vi "Read configuration.vi"(8 "error in":errorcluster, 11 "Multiplexer editor node in":refnum<class "Multiplexer editor node.lvclass">) -> (0 "error out":errorcluster, 2 "configuration":refnum<class "NISE_CEF_serializable configuration.lvclass">, 3 "Multiplexer editor node out":refnum<class "Multiplexer editor node.lvclass">)   [LabVIEW 2021, in "Multiplexer editor node.lvclass"]
uses:
  Multiplexer editor node.lvclass
  <vilib>/NI/Configuration Framework/serializable configuration/NISE_CEF_serializable configuration.lvclass
  Multiplexer editor node.lvclass/Multiplexer editor node.ctl
  configuration/Multiplexer configuration.lvclass
  C:/Program Files (x86)/National Instruments/LabVIEW 2021/vi.lib/NI/Configuration Framework/serializable configuration/NISE_CEF_serializable configuration.lvclass
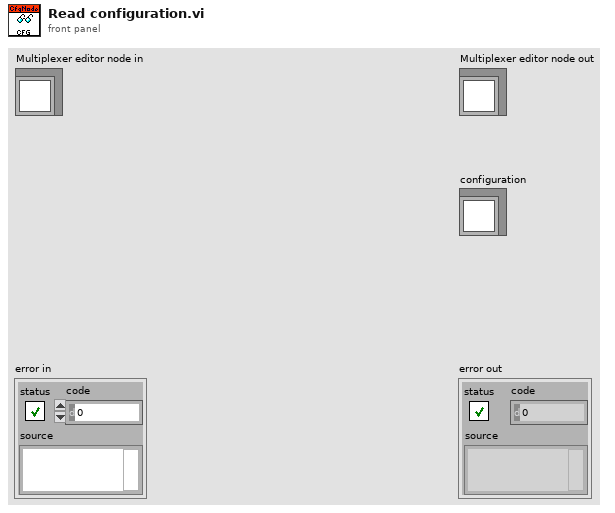
[diagram p1: front panel]
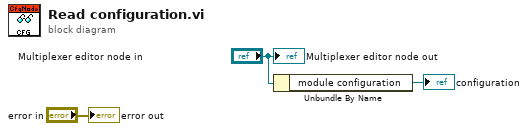
[diagram p0: block diagram]
diagram:
  n1 = Unbundle By Name("Multiplexer editor node in") -> ("module configuration"=→"configuration":refnum<class "Multiplexer configuration.lvclass">)
  "error out" <- "error in"
  "Multiplexer editor node out" <- "Multiplexer editor node in"
